vi "Plot attribute value change event.vi"(5 "Plot ref (target)":refnum<vi>, 7 "top array":refnum<vi>, 8 "PlotRef (event source)":refnum<vi>, 9 "NewAttrib":T1, 10 "OldAttrib":T1, 11 "PlotIdx (target)":i32) -> (0 "error out":errorcluster)   [LabVIEW 2021, in "RocketPlot.lvlib"]
uses:
  RocketPlot.lvlib
  TypeDefs/Plot top row.ctl
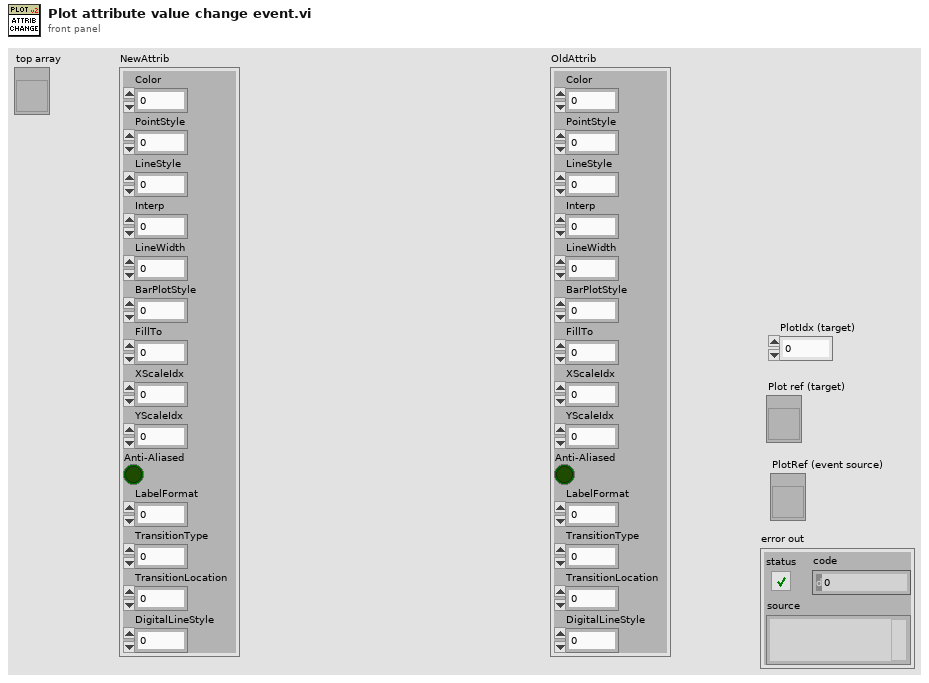
[diagram p1: front panel]
types:
  T1 = cluster{"Color":u32, "PointStyle":u8, "LineStyle":u8, "Interp":u8, "LineWidth":u8, "BarPlotStyle":u8, "FillTo":i16, "XScaleIdx":u32, "YScaleIdx":u32, "Anti-Aliased":bool, "LabelFormat":u8, "TransitionType":u8, "TransitionLocation":u8, "DigitalLineStyle":u8}
  T2 = cluster{"Color":bool, "PointStyle":bool, "LineStyle":bool, "Interp":bool, "LineWidth":bool, "BarPlotStyle":bool, "FillTo":bool, "XScaleIdx":bool, "YScaleIdx":bool, "Anti-Aliased":bool, "LabelFormat":bool, "TransitionType":bool, "TransitionLocation":bool, "DigitalLineStyle":bool}
  T3 = typedef "Plot top row.ctl" = cluster{"PID":string, "index":i32, "PID color":u32, "right axis?":bool, "Flatline?":bool, "Numeric color":u32, "Data":string, "Flat":string}
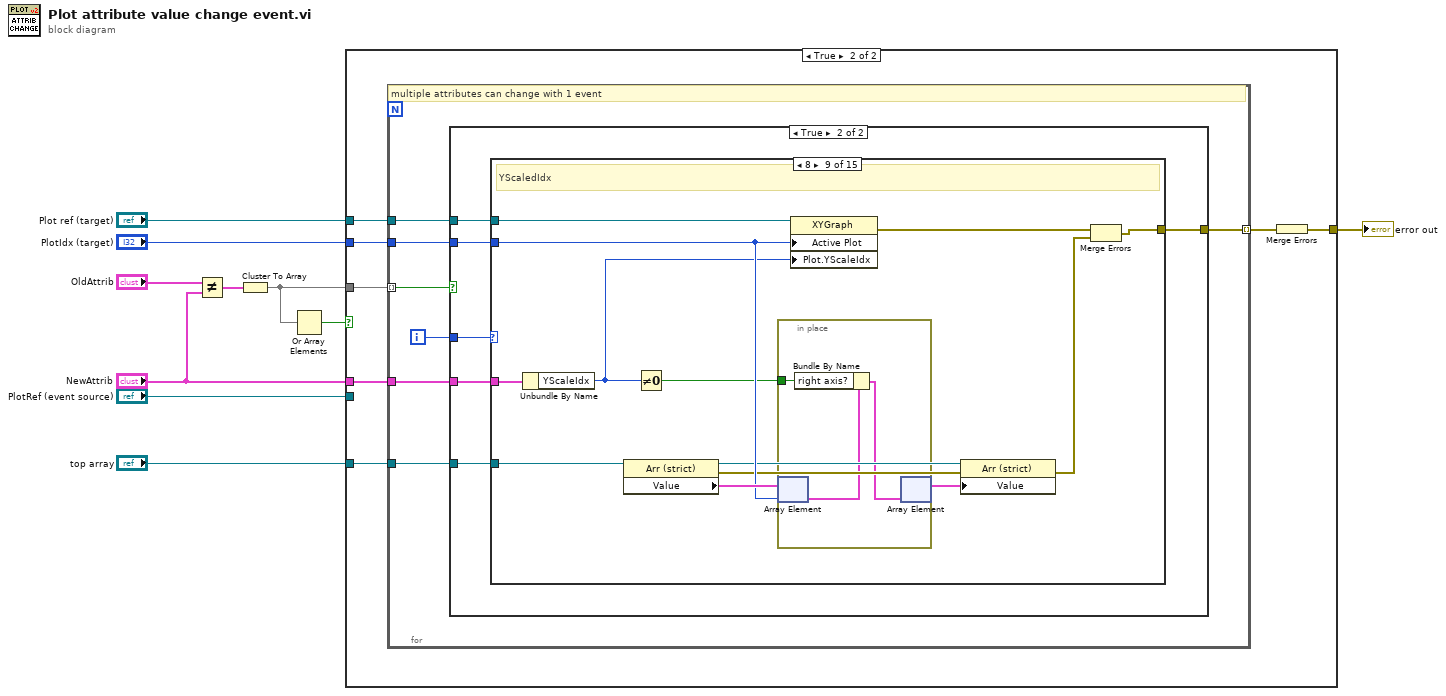
[diagram p0: block diagram]
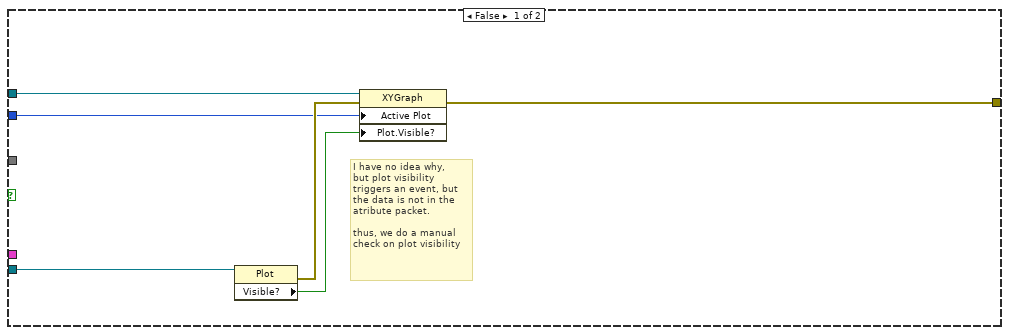
[diagram p2: hidden frame]
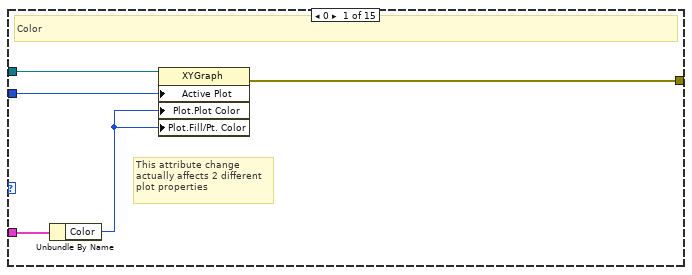
[diagram p4: hidden frame]
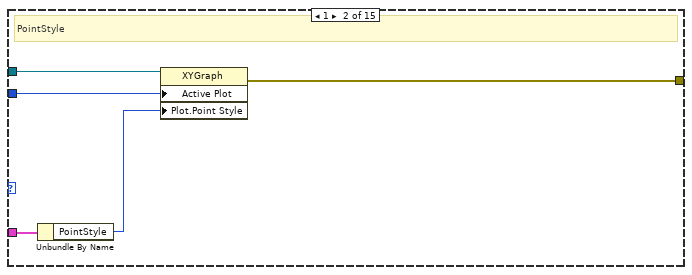
[diagram p5: hidden frame]
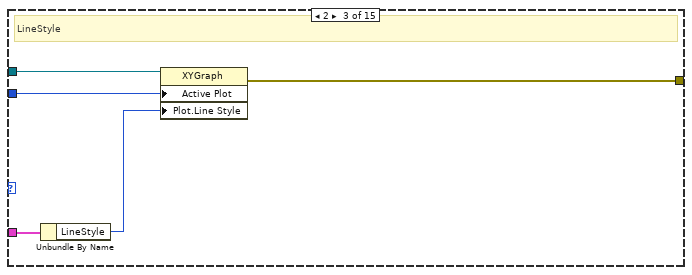
[diagram p6: hidden frame]
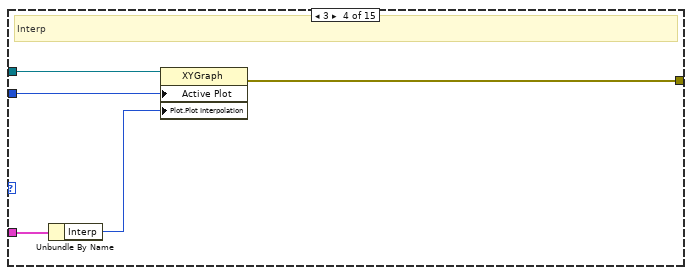
[diagram p7: hidden frame]
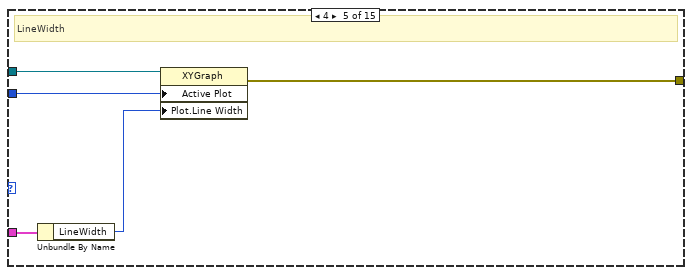
[diagram p8: hidden frame]
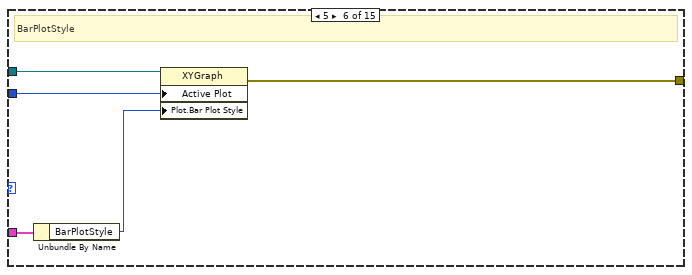
[diagram p9: hidden frame]
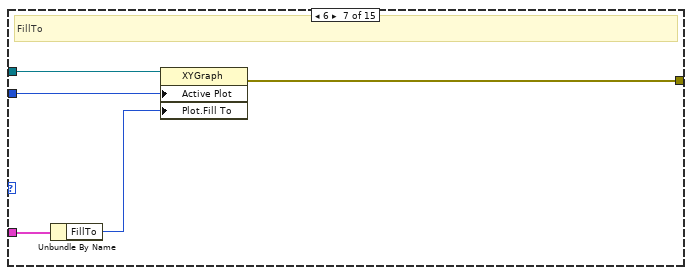
[diagram p10: hidden frame]
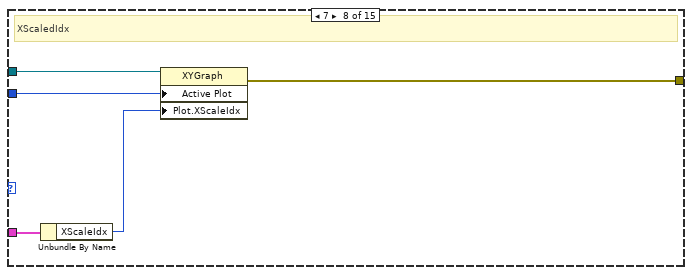
[diagram p11: hidden frame]
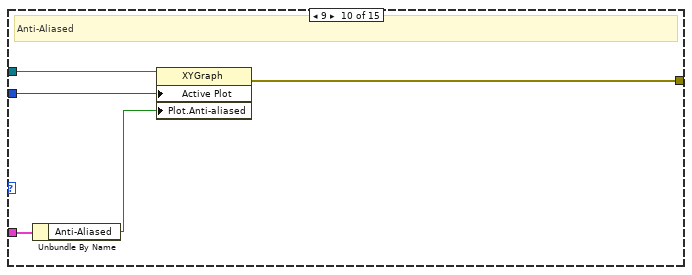
[diagram p12: hidden frame]
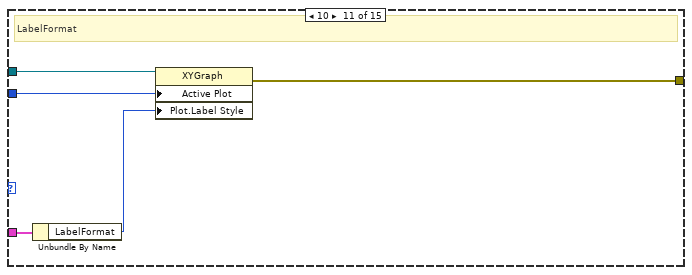
[diagram p13: hidden frame]
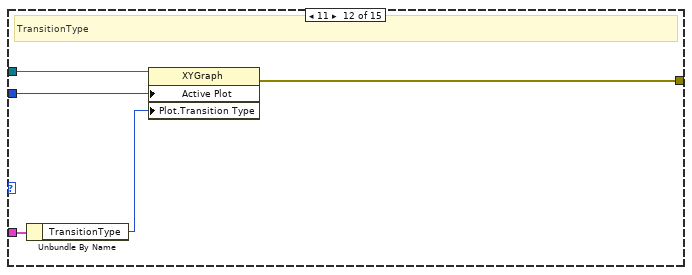
[diagram p14: hidden frame]
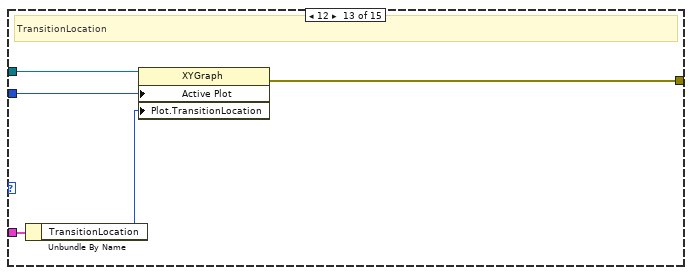
[diagram p15: hidden frame]
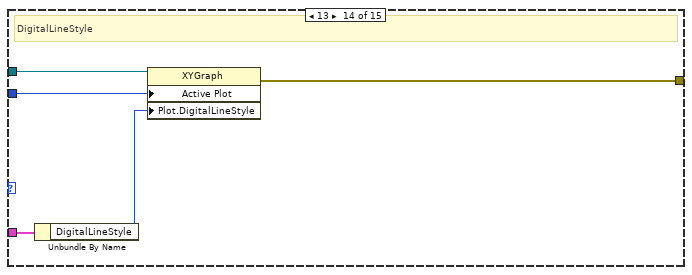
[diagram p16: hidden frame]
diagram:
  n1 = Not Equal?(x="OldAttrib", y="NewAttrib") -> (x != y?=w10:T2)
  n2 = Cluster To Array(cluster=w10) -> (array=w3:bool[])
  n3 = Or Array Elements(Boolean array=w3) -> (logical OR=w2:bool)
  n4 = case shown="True" w2 {
    tunnel: "Plot ref (target)" -> [w14 w23]
    tunnel: "PlotIdx (target)" -> [w13 w22]
    tunnel: "NewAttrib" -> [_ w21]
    tunnel: "PlotRef (event source)" -> [w11 _]
    tunnel: [w12 w17] -> w1
    tunnel: "top array" -> [_ w20]
    tunnel: w3 -> [_ w19]
    frame False {
      # "I have no idea why,\nbut plot visibility\ntriggers an event, but\nthe data is not in the\natribute packet.\n\nthus, we do a manual\ncheck on plot visibility"
      n5 = property class="Plot"(reference=w11) -> (error out=w15:errorcluster, "Visible?"=w16:bool)  [unwired: 1 in, 1 out]
      n6 = property class="XYGraph"(reference=w14, error in=w15, "Active Plot"=w13, "Plot.Visible?"=w16) -> (error out=w12:errorcluster)  [unwired: 1 out]
    }
    frame True {
      n7 = for {
        tunnel: w23 -> [w30]
        tunnel: w22 -> [w29]
        tunnel: w21 -> [w28]
        tunnel: w19 -> [w26] mode=indexing
        tunnel: [w25] -> w18 mode=indexing
        tunnel: w20 -> [w24]
        i -> [w27]
        # "multiple attributes can change with 1 event"
        n8 = case shown="True" w26 {
          tunnel: w30 -> [_ w36]
          tunnel: w29 -> [_ w35]
          tunnel: w28 -> [_ w34]
          tunnel: w27 -> [_ w33]
          tunnel: [_ w32] -> w25
          tunnel: w24 -> [_ w31]
          frame False {
          }
          frame True {
            n9 = case shown="8" w33 {
              tunnel: w34 -> [w40 w45 w50 w55 w60 w65 w70 w75 w88 w96 w101 w106 w111 w116 _]
              tunnel: w36 -> [w41 w46 w51 w56 w61 w66 w71 w76 w89 w97 w102 w107 w112 w117 _]
              tunnel: w35 -> [w39 w44 w49 w54 w59 w64 w69 w74 w85 w95 w100 w105 w110 w115 _]
              tunnel: [w37 w42 w47 w52 w57 w62 w67 w72 w77 w93 w98 w103 w108 w113 _] -> w32
              tunnel: w31 -> [_ _ _ _ _ _ _ _ w87 _ _ _ _ _ _]
              frame 0 {
                # "This attribute change\nactually affects 2 different\nplot properties"
                # "Color"
                n10 = Unbundle By Name(w40) -> ("Color"=w38:u32)
                n11 = property class="XYGraph"(reference=w41, "Active Plot"=w39, "Plot.Plot Color"=w38, "Plot.Fill/Pt. Color"=w38) -> (error out=w37:errorcluster)  [unwired: 1 in, 1 out]
              }
              frame 1 {
                # "PointStyle"
                n12 = Unbundle By Name(w45) -> ("PointStyle"=w43:u8)
                n13 = property class="XYGraph"(reference=w46, "Active Plot"=w44, "Plot.Point Style"=w43) -> (error out=w42:errorcluster)  [unwired: 1 in, 1 out]
              }
              frame 2 {
                # "LineStyle"
                n14 = Unbundle By Name(w50) -> ("LineStyle"=w48:u8)
                n15 = property class="XYGraph"(reference=w51, "Active Plot"=w49, "Plot.Line Style"=w48) -> (error out=w47:errorcluster)  [unwired: 1 in, 1 out]
              }
              frame 3 {
                # "Interp"
                n16 = Unbundle By Name(w55) -> ("Interp"=w53:u8)
                n17 = property class="XYGraph"(reference=w56, "Active Plot"=w54, "Plot.Plot Interpolation"=w53) -> (error out=w52:errorcluster)  [unwired: 1 in, 1 out]
              }
              frame 4 {
                # "LineWidth"
                n18 = Unbundle By Name(w60) -> ("LineWidth"=w58:u8)
                n19 = property class="XYGraph"(reference=w61, "Active Plot"=w59, "Plot.Line Width"=w58) -> (error out=w57:errorcluster)  [unwired: 1 in, 1 out]
              }
              frame 5 {
                # "BarPlotStyle"
                n20 = Unbundle By Name(w65) -> ("BarPlotStyle"=w63:u8)
                n21 = property class="XYGraph"(reference=w66, "Active Plot"=w64, "Plot.Bar Plot Style"=w63) -> (error out=w62:errorcluster)  [unwired: 1 in, 1 out]
              }
              frame 6 {
                # "FillTo"
                n22 = Unbundle By Name(w70) -> ("FillTo"=w68:i16)
                n23 = property class="XYGraph"(reference=w71, "Active Plot"=w69, "Plot.Fill To"=w68) -> (error out=w67:errorcluster)  [unwired: 1 in, 1 out]
              }
              frame 7 {
                # "XScaledIdx"
                n24 = Unbundle By Name(w75) -> ("XScaleIdx"=w73:u32)
                n25 = property class="XYGraph"(reference=w76, "Active Plot"=w74, "Plot.XScaleIdx"=w73) -> (error out=w72:errorcluster)  [unwired: 1 in, 1 out]
              }
              frame 8 {
                # "YScaledIdx"
                n26 = Unbundle By Name(w88) -> ("YScaleIdx"=w84:u32)
                n27 = property class="Arr (strict)"(reference=w87) -> (reference out=w82:refnum<vi>, error out=w81:errorcluster, "Value"=w86:T3[])  [unwired: 1 in]
                n28 = Not Equal To 0?(x=w84) -> (x != 0?=w83:bool)
                n29 = in-place {
                  in-place-border: w83 -> [w91]
                  n30 = in-place-array #1(w86, w85) -> (w92:T3)
                  n31 = Bundle By Name(cluster=w92, "right axis?"=w91) -> (w90:T3)
                  n32 = in-place-array #1(w90) -> (w80:T3[])  [unwired: 1 out]
                }
                n33 = property class="XYGraph"(reference=w89, "Active Plot"=w85, "Plot.YScaleIdx"=w84) -> (error out=w79:errorcluster)  [unwired: 1 in, 1 out]
                n34 = property class="Arr (strict)"(reference=w82, error in=w81, "Value"=w80) -> (error out=w78:errorcluster)  [unwired: 1 out]
                n35 = Merge Errors(w79, w78) -> (w77:errorcluster)
              }
              frame 9 {
                # "Anti-Aliased"
                n36 = Unbundle By Name(w96) -> ("Anti-Aliased"=w94:bool)
                n37 = property class="XYGraph"(reference=w97, "Active Plot"=w95, "Plot.Anti-aliased"=w94) -> (error out=w93:errorcluster)  [unwired: 1 in, 1 out]
              }
              frame 10 {
                # "LabelFormat"
                n38 = Unbundle By Name(w101) -> ("LabelFormat"=w99:u8)
                n39 = property class="XYGraph"(reference=w102, "Active Plot"=w100, "Plot.Label Style"=w99) -> (error out=w98:errorcluster)  [unwired: 1 in, 1 out]
              }
              frame 11 {
                # "TransitionType"
                n40 = Unbundle By Name(w106) -> ("TransitionType"=w104:u8)
                n41 = property class="XYGraph"(reference=w107, "Active Plot"=w105, "Plot.Transition Type"=w104) -> (error out=w103:errorcluster)  [unwired: 1 in, 1 out]
              }
              frame 12 {
                # "TransitionLocation"
                n42 = Unbundle By Name(w111) -> ("TransitionLocation"=w109:u8)
                n43 = property class="XYGraph"(reference=w112, "Active Plot"=w110, "Plot.TransitionLocation"=w109) -> (error out=w108:errorcluster)  [unwired: 1 in, 1 out]
              }
              frame 13 {
                # "DigitalLineStyle"
                n44 = Unbundle By Name(w116) -> ("DigitalLineStyle"=w114:u8)
                n45 = property class="XYGraph"(reference=w117, "Active Plot"=w115, "Plot.DigitalLineStyle"=w114) -> (error out=w113:errorcluster)  [unwired: 1 in, 1 out]
              }
              frame Default {
              }
            }
          }
        }
      }
      n46 = Merge Errors(w18) -> (w17:errorcluster)
    }
  }
  "error out" <- w1
